vi "test Set ObjectType_1.vi"(11 "Test Case In":refnum<class "test EDS.lvclass">) -> (0 "error out":errorcluster, 3 "Test Case Out":refnum<class "test EDS.lvclass">)   [LabVIEW 2024, in "test EDS.lvclass"]
uses:
  test EDS.lvclass
  C:/Program Files/National Instruments/LabVIEW 2024/vi.lib/Astemes/LUnit/Test Case.lvclass
  <vilib>/PNR/JSONtext Object Serialization/Generic Object Serializer/Generic Object Serializer.lvclass
  C:/Program Files/National Instruments/LabVIEW 2024/vi.lib/JDP Science/JSONtext/LVClass Serializer/JSONtext LVClass Serializer.lvclass
  <vilib>/PNR/JSONtext Object Serialization/Generic Object Serializer/Type Name Handling.ctl
  Core/Object Type/Object Type Base.lvclass
  <vilib>/PNR/JSONtext Object Serialization/Generic Object Serializer/Generic Object Serializer.lvclass/Generic Object Serializer.ctl
  <vilib>/Astemes/LUnit/Test Case.lvclass/Test Case.ctl
  bdd25f00-0f07-479c-b713-0b173a884aa2.vi
  d0c0fd45-a26b-4681-8f26-a028a3b3cd1b.vi
  4993e8ee-a06a-463a-9684-69129f64d5ce.vi
  <vilib>/PNR/JSONtext Object Serialization/Generic Object Serializer/Write Type Name Handling.vi
  <vilib>/JDP Science/JSONtext/Find Item.vi
  <vilib>/Astemes/LUnit/Append Pass Result.vi
  <vilib>/Astemes/LUnit/Append Fail Result.vi
  <vilib>/Astemes/LUnit/Describe Comparison.vi
  4993e8ee-a06a-463a-9684-69129f64d5ce.vi/9c5d11cd-9439-4240-a1ee-d9baace9c924.vi
  <vilib>/JDP Science/JSONtext/Next JSON Value.vi
  <vilib>/JDP Science/JSONtext/String Subset.vi
  <vilib>/Astemes/LUnit/Run In UI.vi
  <vilib>/JDP Science/JSONtext/Parsing/Advance past next JSON Value (inlined COPY).vi
  <vilib>/Utility/error.llb/Clear Errors.vi
  <vilib>/JDP Science/JSONtext/Parsing/Advance past whitespace.vi
  <vilib>/JDP Science/JSONtext/Parsing/Advance past String.vi
  <vilib>/JDP Science/JSONtext/Parsing/Advance past Number.vi
  <vilib>/JDP Science/JSONtext/Parsing/Advance past Line Ending.vi
  <vilib>/JDP Science/JSONtext/Variant to JSON Text.vi
  <vilib>/JDP Science/JSONtext/Parsing/Parse Full Path or Item Name.vi
  <vilib>/JDP Science/JSONtext/Parsing/Advance past Array.vi
  <vilib>/JDP Science/JSONtext/Parsing/Advance past Object.vi
  <vilib>/JDP Science/JSONtext/support/Error Cluster From Code.vi
  <vilib>/JDP Science/JSONtext/Offset/Find Item Locations by Path.vi
  <vilib>/JDP Science/JSONtext/JSON text to Variant.vi
  <vilib>/Astemes/LUnit/Describe Variant.vi
  <vilib>/JDP Science/JSONtext/LVClass Serializer/JSONtext LVClass Serializer.lvclass
  Core/Value/Value.lvclass
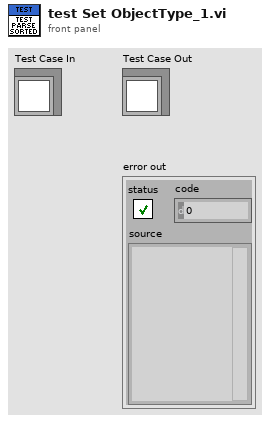
[diagram p1: front panel]
types:
  T1 = typedef "Generic Object Serializer.lvclass/Type Name Handling.ctl" = enum16{"None", "Inline"}
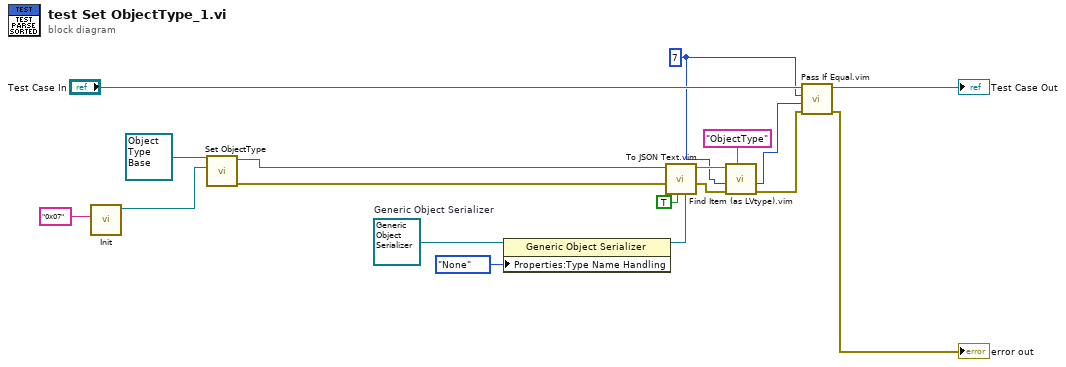
[diagram p0: block diagram]
diagram:
  w1 = u8 7
  w15 = refnum<class "Generic Object Serializer.lvclass"> refnum  # Generic Object Serializer
  n1 = call "Init.vi"("Value"="0x07") -> ("Value out"=w10:refnum<class "Value.lvclass">)  [unwired: 9 in, 1 out]
  n2 = call-dynamic "Set ObjectType.vi"("ObjectType"=w10, "Object Type in"=refnum<class "Object Type Base.lvclass"> refnum ("EDS.lvlib:Object Type.lvclass")) -> ("error out"=w7:errorcluster, "Object Type out"=w8:refnum<class "Object Type Base.lvclass">)  [unwired: 8 in]
  n3 = property class="Generic Object Serializer"(reference=w15, "Properties:Type Name Handling"=Type_Name_Handling."None" ("Type Name Handling")) -> (reference out=w14:refnum<class "Generic Object Serializer.lvclass">)  [unwired: 1 in, 1 out]
  n4 = call "To JSON Text.vim"("LVClass Serializer"=w14, "Pretty Print?"=TRUE, "error in (no error)"=w7, "Anything"=w8) -> ("error out"=w3:errorcluster, "<JSON>"=w4:string)  [unwired: 6 in]
  n5 = call "Find Item (as LVtype).vim"("$Path or Item Name"="ObjectType", "error in (no error)"=w3, "Data Type and Default Value"=w1, "JSON"=w4) -> ("error out"=w2:errorcluster, "Data"=w5:u8)  [unwired: 4 in, 2 out]
  n6 = call "Pass If Equal.vim"("error in (no error)"=w2, "Actual"=w5, "Expected"=w1, "LUnit Test Case In"="Test Case In") -> ("error out"=→"error out":errorcluster, "LUnit Test Case Out"=→"Test Case Out":refnum<class "test EDS.lvclass">)  [unwired: 6 in]
